vi "Count.vi"(7 "Chess board":T1) -> (6 "BlackNum":u16, 10 "WhiteNum":u16)   [LabVIEW 2009]
doc: "Count the chess board. Return the munber of the black and white stones."
uses:
  Controls/Chess.ctl
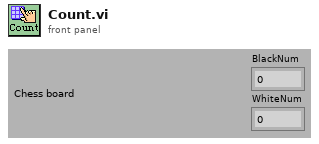
[diagram p1: front panel]
types:
  T1 = typedef "Chess.ctl" = u16[][]
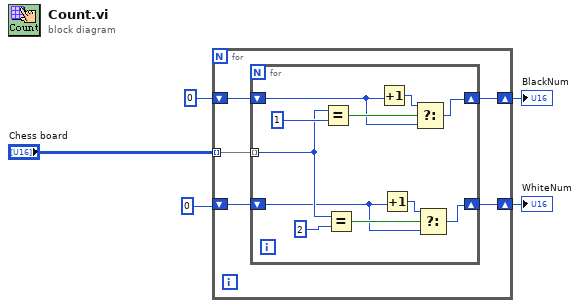
[diagram p0: block diagram]
diagram:
  n1 = for {
    tunnel: "Chess board" -> [w10] mode=indexing
    shift-right: [w8] -> w2
    shift-left: u16 0 ("y") -> [w9]
    shift-right: [w6] -> w1
    shift-left: u16 0 ("y") -> [w7]
    n2 = for {
      tunnel: w10 -> [w12] mode=indexing
      shift-right: [w17] -> w8
      shift-left: w9 -> [w18]
      shift-right: [w13] -> w6
      shift-left: w7 -> [w11]
      n3 = Equal?(x=w12, y=u16 1) -> (x = y?=w21:bool)
      n4 = Equal?(x=w12, y=u16 2) -> (x = y?=w14:bool)
      n5 = Increment(x=w18) -> (x+1=w19:u16)
      n6 = Increment(x=w11) -> (x+1=w16:u16)
      n7 = Select(t=w19, s=w21, f=w18) -> (s? t:f=w17:u16)
      n8 = Select(t=w16, s=w14, f=w11) -> (s? t:f=w13:u16)
    }
  }
  "BlackNum" <- w2
  "WhiteNum" <- w1
